vi "ATSpectrograph_getResponse_homeLinearStage.vi"(8 "error in (no error)":errorcluster, 11 "ackcmd_Ctl":T1={"cmdSeqNum"=0, "ack"=0, "error"=0, "result"="                                                                                                                                                                                                                                                                "}) -> (0 "error out":errorcluster, 2 "function return":i32, 3 "ackcmd_Ctl out":T1={"cmdSeqNum"=0, "ack"=0, "error"=0, "result"="                                                                                                                                                                                                                                                                "})   [LabVIEW 2016, in "SALLV_ATSpectrograph.lvlib"]
doc: "int ATSpectrograph_shm_getResponse_homeLinearStageLV(ATSpectrograph_ackcmdLV *ackcmd_Ctl);"
uses:
  SALLV_ATSpectrograph.lvlib
  DataTypes/ackcmd.ctl
  SALLV_ATSpectrograph.so
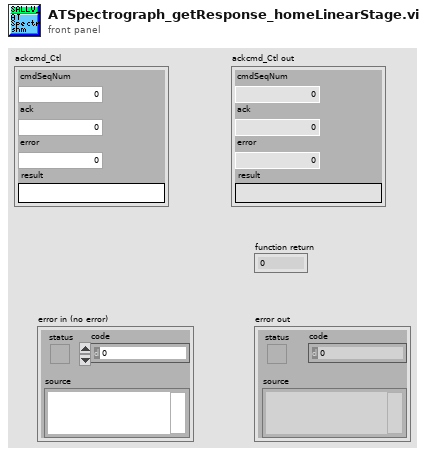
[diagram p1: front panel]
types:
  T1 = typedef "SALLV_ATSpectrograph.lvlib/ackcmd.ctl" = cluster{"cmdSeqNum":i32, "ack":i32, "error":i32, "result":string}
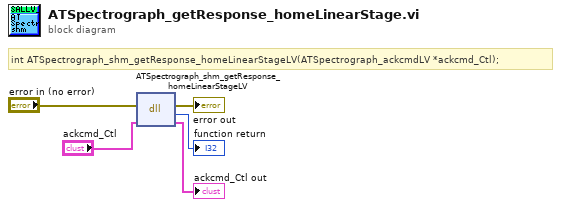
[diagram p0: block diagram]
diagram:
  # "int ATSpectrograph_shm_getResponse_homeLinearStageLV(ATSpectrograph_ackcmdLV *ackcmd_Ctl);"
  n1 = dll-call lib="home/harini/tcs/SALLV_ATSpectrograph/SALLV_ATSpectrograph.*" fn="ATSpectrograph_shm_getResponse_homeLinearStageLV"(error in="error in (no error)", "ackcmd_Ctl"="ackcmd_Ctl") -> (error out=→"error out":errorcluster, →"function return":i32, "ackcmd_Ctl"=→"ackcmd_Ctl out":T1)  [unwired: 2 in, 1 out]
